vi "MS-Word Property Node.vi"   [LabVIEW 2017, in "LabVIEW NPOI.lvlib" / "MS-Word.lvclass"]
uses:
  MS-Word.lvclass
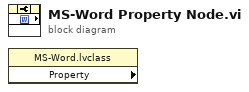
[diagram p0: block diagram]
diagram:
  n1 = property class="MS-Word.lvclass" props=[]() -> ()  [unwired: 2 in, 3 out]
